vi "MathCad_Wrkshts_Close.vi"(8 "error in":errorcluster, 11 "Worksheets Reference":refnum<k7>) -> (0 "error out":errorcluster)   [LabVIEW 2015]
doc: "Closes the reference to the Worksheets Class that was opened by the Mathcad_File_Open.vi.\n\nInputs-\nWorksheets Reference- Reference to the Worksheets Class. This has to be closed after the Worksheet Reference."
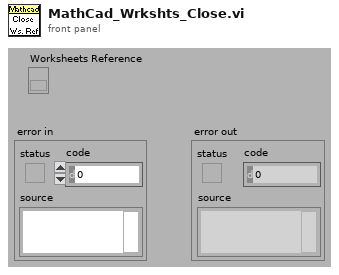
[diagram p1: front panel]
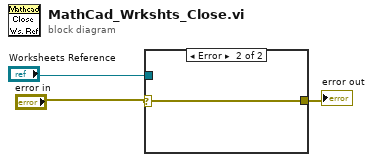
[diagram p0: block diagram]
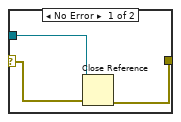
[diagram p2: hidden frame]
diagram:
  n1 = case shown="Error" "error in" {
    selector: "error in" -> [w4 w7]
    tunnel: "Worksheets Reference" -> [w6 _]
    tunnel: [w5 w7] -> w2
    frame No Error {
      n2 = Close Reference(reference=w6, error in (no error)=w4) -> (error out=w5:errorcluster)
    }
    frame Error {
    }
  }
  "error out" <- w2
